vi "BB_Check_Gyro_Direction.vi"() -> (3 "chgDirection":bool)   [LabVIEW 2012]
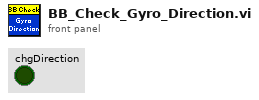
[diagram p1: front panel]
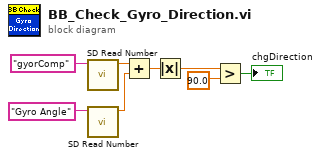
[diagram p0: block diagram]
diagram:
  n1 = call <vilib>:"SD Read Number.vi"("Name"="gyorComp") -> ("Numeric"=w2:dbl)  [unwired: 8 in, 2 out]
  n2 = call <vilib>:"SD Read Number.vi"("Name"="Gyro Angle") -> ("Numeric"=w5:dbl)  [unwired: 8 in, 2 out]
  n3 = Add(x=w2, y=w5) -> (x+y=w4:dbl)
  n4 = Absolute Value(x=w4) -> (abs(x)=w7:dbl)
  n5 = Greater?(x=w7, y=90.0) -> (0:→"chgDirection":bool)
